vi "CalcTargetError.vi"(11 "Chosen Target":T1) -> (2 "Y Error (Degrees)":dbl, 3 "X Error (Degrees)":dbl)   [LabVIEW 2011]
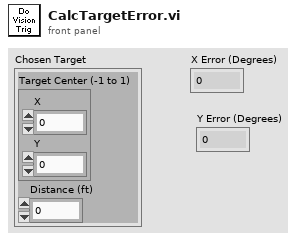
[diagram p1: front panel]
types:
  T1 = cluster{"Target Center (-1 to 1)":cluster{"X":dbl, "Y":dbl}, "Distance (ft)":dbl}
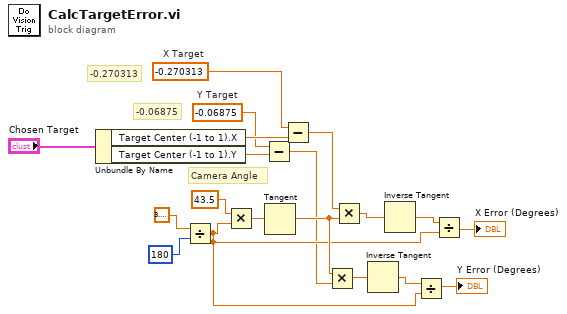
[diagram p0: block diagram]
diagram:
  w2 = -0.270313  # X Target
  w1 = -0.06875  # Y Target
  # "-0.06875"
  # "-0.270313"
  # "Camera Angle"
  n1 = Unbundle By Name("Chosen Target") -> ("Target Center (-1 to 1).X"=w5:dbl, "Target Center (-1 to 1).Y"=w4:dbl)
  n2 = Divide(x=3.141592653589793, y=180) -> (x/y=w8:dbl)
  n3 = Multiply(x=43.5, y=w8) -> (x*y=w15:dbl)
  n4 = Subtract(x=w1, y=w4) -> (x-y=w3:dbl)
  n5 = Tangent(1:w15) -> (0:w9:dbl)
  n6 = Subtract(x=w2, y=w5) -> (x-y=w6:dbl)
  n7 = Multiply(x=w9, y=w3) -> (x*y=w10:dbl)
  n8 = Multiply(x=w6, y=w9) -> (x*y=w14:dbl)
  n9 = Inverse Tangent(1:w10) -> (0:w11:dbl)
  n10 = Inverse Tangent(1:w14) -> (0:w13:dbl)
  n11 = Divide(x=w11, y=w8) -> (x/y=→"Y Error (Degrees)":dbl)
  n12 = Divide(x=w13, y=w8) -> (x/y=→"X Error (Degrees)":dbl)
